vi "test_get_rt_status.vi"() -> ()   [LabVIEW 2019]
uses:
  <vilib>/Utility/error.llb/DialogType.ctl
panel:
  in  "address":string="139.229.170.56"
  out "log":string
  out "json error":errorcluster
  out "data":refnum<queue>
  out "error out":errorcluster
  out "data out":string="{\"time\":\"2025-03-18T13:53:58.728Z\",\"hostComms\":false,\"topBoxComms\":true,\"AZPos\":0.43617177754640579224,\"AZPosReq\":0,\"AZPosError\":0,\"AZEncCounts\":82268427657,\"AZEncStatus\":1025,\"AZLastRot\":\"reverse\",\"mode\":\"stop\",\"modeReq\":\"stop\",\"subMode\":0,\"cmd\":0,\"buttons\":{\"EMStop\":false,\"forward\":false,\"reverse\":false,\"open\":false,\"close\":false,\"up\":false,\"down\":false,\"forceStop\":false},\"envSensor\":false,\"homed\":true,\"homing\":false,\"homeSensor\":false,\"config\":{\"cloudEn\":false,\"AZEncNeg\":false,\"AZEncRef\":86281702555,\"AZEncStep\":4018143232,\"homePos\":0,\"AZTimeout\":120000,\"AZEncNoError\":1025,\"posHSThreshold\":5.0000000372529029846,\"posTol\":0.4999999701976776123,\"cloudTimeout\":5000,\"revDly\":4000,\"AZEncCenter\":68719476735,\"AZEncCenterThreshold\":55807545,\"AZEncCenterTol\":5580754,\"watchdogTim\":600,\"autoShutEn\":true,\"antWifi\":true},\"errors\":{\"EMStop\":false,\"AZEnc\":false,\"AZTimeout\":false,\"cloud\":false,\"M1\":false,\"M2\":false,\"M4\":false,\"watchdogTime\":true,\"shutdown\":true},\"logs\":{\"time\":[],\"messages\":[]}}"
  in  "stop":bool
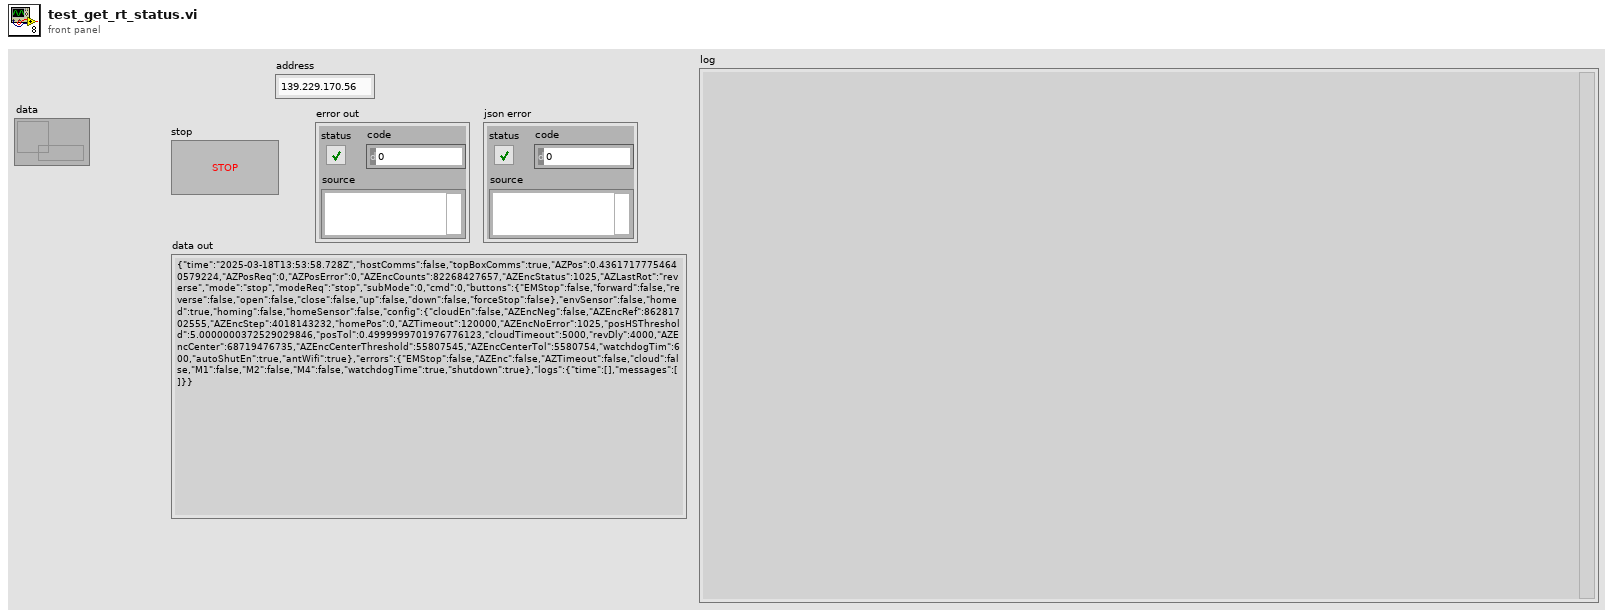
[diagram p1: front panel]
types:
  T1 = cluster{"time":string, "hostComms":bool, "topBoxComms":bool, "AZPos":dbl, "AZPosReq":dbl, "AZPosError":dbl, "AZEncCounts":u64, "AZEncStatus":u16, "AZLastRot":string, "mode":string, "modeReq":string, "subMode":u8, "cmd":i8, "buttons":cluster{"EMStop":bool, "forward":bool, "reverse":bool, "open":bool, "close":bool, "up":bool, "down":bool, "forceStop":bool}, "envSensor":bool, "homed":bool, "homing":bool, "homeSensor":bool, "config":cluster{"cloudEn":bool, "AZEncNeg":bool, "AZEncRef":u64, "AZEncStep":u64, "homePos":dbl, "AZTimeout":u32, "AZEncNoError":u16, "posHSThreshold":dbl, "posTol":dbl, "cloudTimeout":u32, "revDly":u32, "AZEncCenter":u64, "AZEncCenterThreshold":u64, "AZEncCenterTol":u64, "watchdogTim":i32, "autoShutEn":bool, "antWifi":bool}, "errors":cluster{"EMStop":bool, "AZEnc":bool, "AZTimeout":bool, "cloud":bool, "M1":bool, "M2":bool, "M4":bool, "watchdogTime":bool, "shutdown":bool}, "logs":cluster{"time":string[], "messages":string[]}}
  T2 = enum16{"Standard", "Buffered", "CRLF", "Immediate"}
  T3 = typedef "DialogType.ctl" = u16
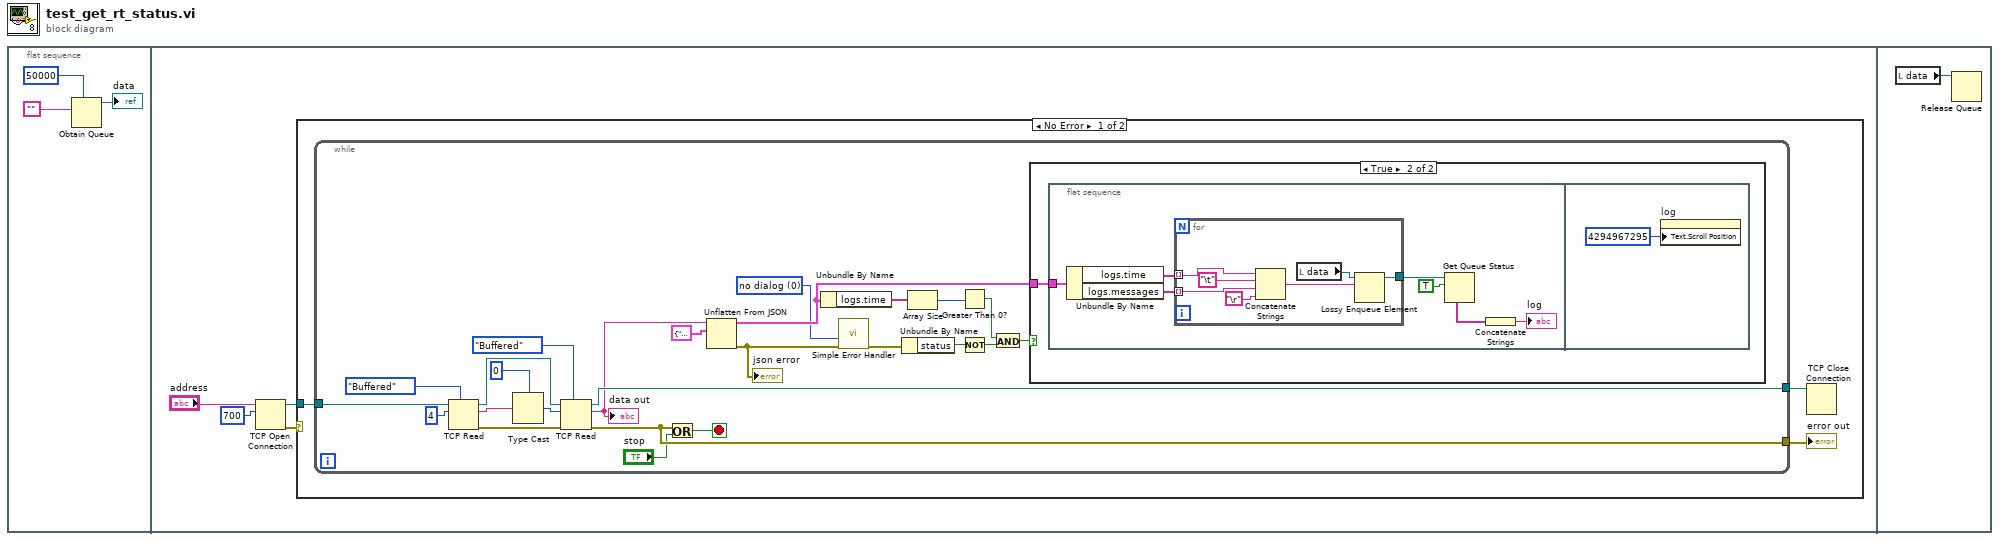
[diagram p0: block diagram]
diagram:
  n1 = flat-sequence {
    frame #0 {
      n2 = Obtain Queue(max queue size (-1, unlimited)=50000, element data type="") -> (queue out=→"data":refnum<queue>)  [unwired: 3 in, 2 out]
    }
    frame #1 {
      n3 = TCP Open Connection(address="address", remote port or service name=u16 700) -> (connection ID=w4:refnum<k5>, error out=w5:errorcluster)  [unwired: 3 in]
      n4 = case shown="No Error" w5 {
        tunnel: w4 -> [w10 _]
        frame No Error {
          n5 = while {
            tunnel: w10 -> [w35]
            tunnel: [w30] -> w8
            tunnel: [w29] -> w9
            stop <- w31 stop-if-true
            w11 = T3 0 items=["no dialog", "OK message", "continue or stop message", "OK message + warnings", "continue/stop + warnings"] ("type of dialog (OK msg:1)")
            n6 = TCP Read(connection ID=w35, bytes to read=4, 7:T2."Buffered" ("mode (standard)")) -> (connection ID out=w33:refnum<k5>, data out=w25:string, error out=w32:errorcluster)  [unwired: 2 in]
            n7 = Type Cast(type=0 ("length"), x=w25) -> (*(type *) &x=w24:i32)
            n8 = TCP Read(connection ID=w33, bytes to read=w24, error in (no error)=w32, 7:T2."Buffered" ("mode (standard)")) -> (connection ID out=w30:refnum<k5>, data out=w22:string, error out=w29:errorcluster)  [unwired: 1 in]
            "data out" <- w22
            n9 = Or(x=w29, y="stop") -> (x .or. y?=w31:bool)
            n10 = Unflatten From JSON(JSON string=w22, type and defaults=T1 {"time"="", "hostComms"=FALSE, "topBoxComms"=FALSE, "AZPos"=0.0, "AZPosReq"=0.0, "AZPosError"=0.0, "AZEncCounts"=0, "AZEncStatus"=0, "AZLastRot"="", "mode"="", "modeReq"="", "subMode"=0, "cmd"=0, "buttons"={"EMStop"=FALSE, "forward"=FALSE, "reverse"=FALSE, "open"=FALSE, "close"=FALSE, "up"=FALSE, "down"=FALSE, "forceStop"=FALSE}, "envSensor"=FALSE, "homed"=FALSE, "homing"=FALSE, "homeSensor"=FALSE, "config"={"cloudEn"=FALSE, "AZEncNeg"=FALSE, "AZEncRef"=0, "AZEncStep"=0, "homePos"=0.0, "AZTimeout"=0, "AZEncNoError"=0, "posHSThreshold"=0.0, "posTol"=0.0, "cloudTimeout"=0, "revDly"=0, "AZEncCenter"=0, "AZEncCenterThreshold"=0, "AZEncCenterTol"=0, "watchdogTim"=0, "autoShutEn"=FALSE, "antWifi"=FALSE}, "errors"={"EMStop"=FALSE, "AZEnc"=FALSE, "AZTimeout"=FALSE, "cloud"=FALSE, "M1"=FALSE, "M2"=FALSE, "M4"=FALSE, "watchdogTime"=FALSE, "shutdown"=FALSE}, "logs"={"time"=[], "messages"=[]}} ("output cluster")) -> (value=w18:T1, error out=w13:errorcluster)  [unwired: 5 in]
            "json error" <- w13
            n11 = Unbundle By Name(w18) -> ("logs.time"=w17:string[])
            n12 = call <vilib>:"Simple Error Handler.vi"("type of dialog (OK msg:1)"=w11, "error in (no error)"=w13) -> ("error out"=w12:errorcluster)  [unwired: 3 in, 4 out]
            n13 = Unbundle By Name(w12) -> ("status"=w20:bool)
            n14 = Array Size(array=w17) -> (size(s)=w16:i32)
            n15 = Greater Than 0?(x=w16) -> (x > 0?=w15:bool)
            n16 = Not(x=w20) -> (.not. x?=w19:bool)
            n17 = And(x=w15, y=w19) -> (x .and. y?=w14:bool)
            n18 = case shown="True" w14 {
              tunnel: w18 -> [_ w36]
              frame False {
              }
              frame True {
                n19 = flat-sequence {
                  tunnel: w36 -> [w43]
                  frame #0 {
                    n20 = Unbundle By Name(w43) -> ("logs.time"=w42:string[], "logs.messages"=w41:string[])
                    n21 = for {
                      tunnel: w42 -> [w48] mode=indexing
                      tunnel: w41 -> [w47] mode=indexing
                      tunnel: [w44] -> w40
                      n22 = Concatenate Strings(w48, "\t", w47, "\r") -> (w45:string)
                      n23 = local read "data"() -> (w46:refnum<queue>)
                      n24 = Lossy Enqueue Element(queue=w46, element=w45) -> (queue out=w44:refnum<queue>)  [unwired: 1 in, 3 out]
                    }
                    n25 = Get Queue Status(queue=w40, return elements? (F)=TRUE) -> (elements=w38:string[])  [unwired: 1 in, 7 out]
                    n26 = Concatenate Strings(w38) -> (→"log":string)
                  }
                  frame #1 {
                    n27 = property on="log" class="Str"("Text.Scroll Position"=u32 4294967295) -> ()  [unwired: 2 in, 2 out]
                  }
                }
              }
            }
          }
          "error out" <- w9
          n28 = TCP Close Connection(connection ID=w8) -> ()  [unwired: 2 in, 2 out]
        }
        frame Error {
        }
      }
    }
    frame #2 {
      n29 = local read "data"() -> (w52:refnum<queue>)
      n30 = Release Queue(queue=w52) -> ()  [unwired: 2 in, 3 out]
    }
  }
